vi "Optical Pulse Sequence Generator with ref pulse.vi"(6 "N Loop":i32=25000, 7 "Sig/Ref pause":dbl, 8 "AOM Rest time":dbl, 9 "Signal delay":dbl, 10 "APD signal width":dbl, 11 "AOM Pulse length":dbl=3e-07) -> (0 "Array":T1(array[cluster]), 3 "No. Instructions":i32)   [LabVIEW 2012]
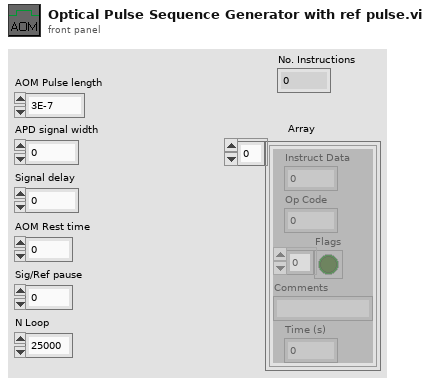
[diagram p1: front panel]
types:
  T1 = cluster{"Instruct Data":i32, "Op Code":i32, "Flags":bool[], "Comments":string, "Time (s)":dbl}[]
  T2 = cluster{"Instruct Data":i32, "Op Code":i32, "Flags":bool[], "Comments":string, "Time (s)":dbl}
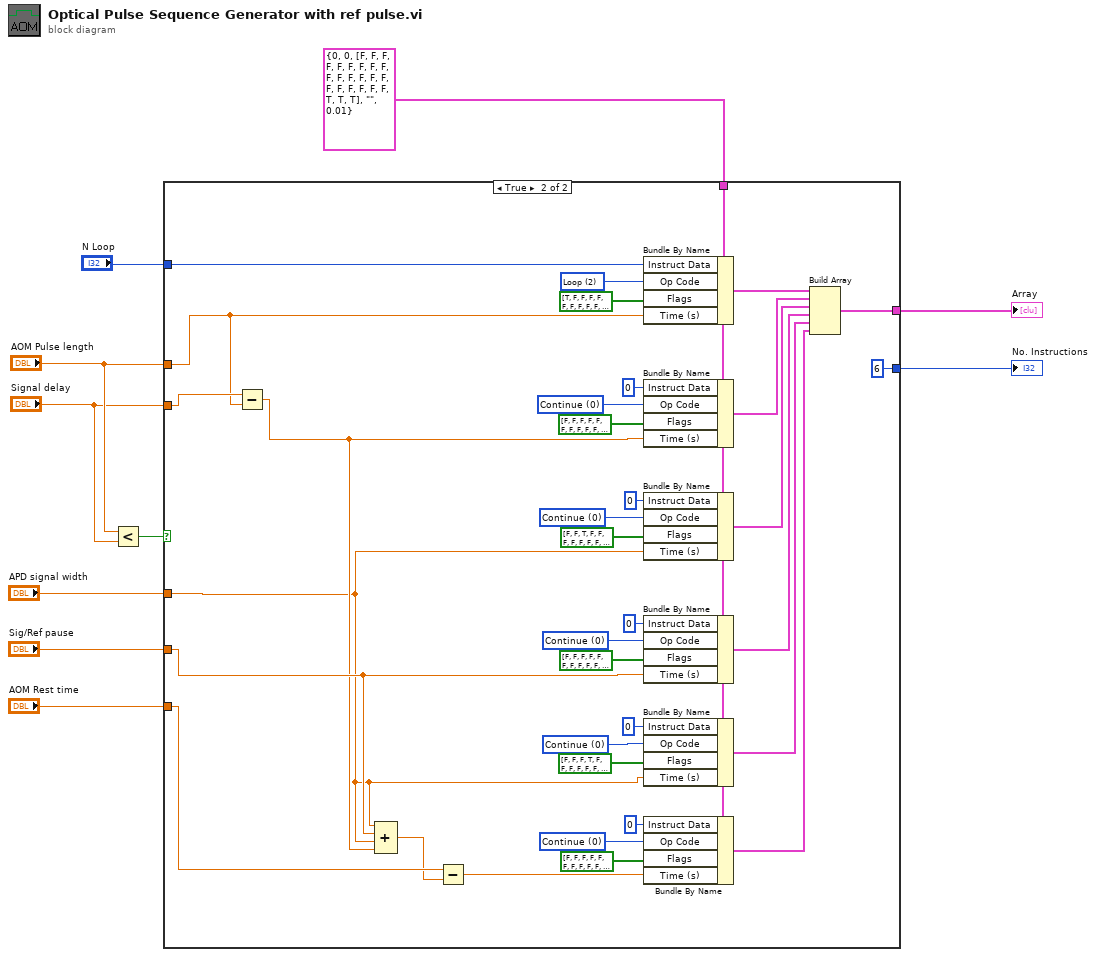
[diagram p0: block diagram]
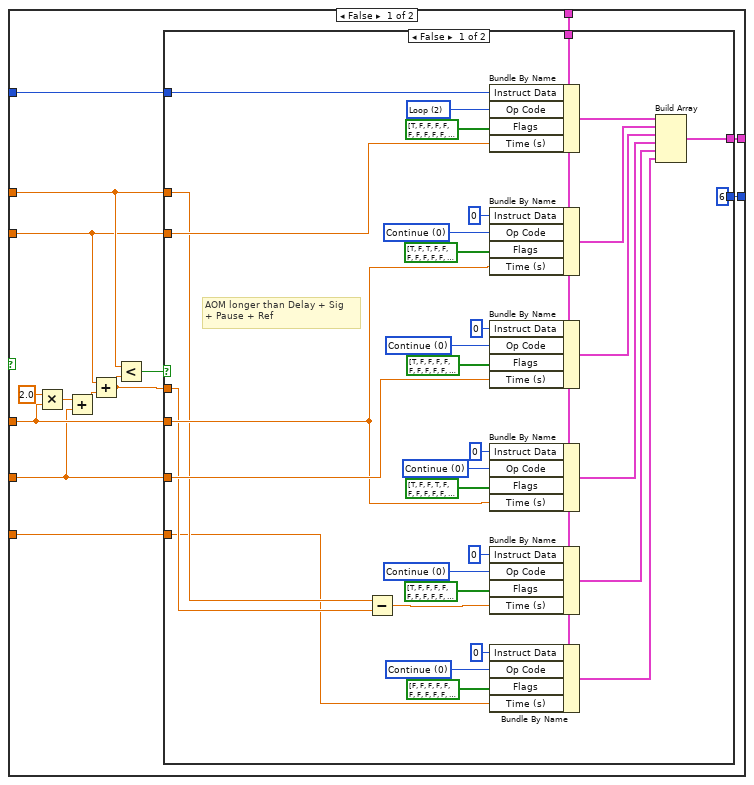
[diagram p2: hidden frame]
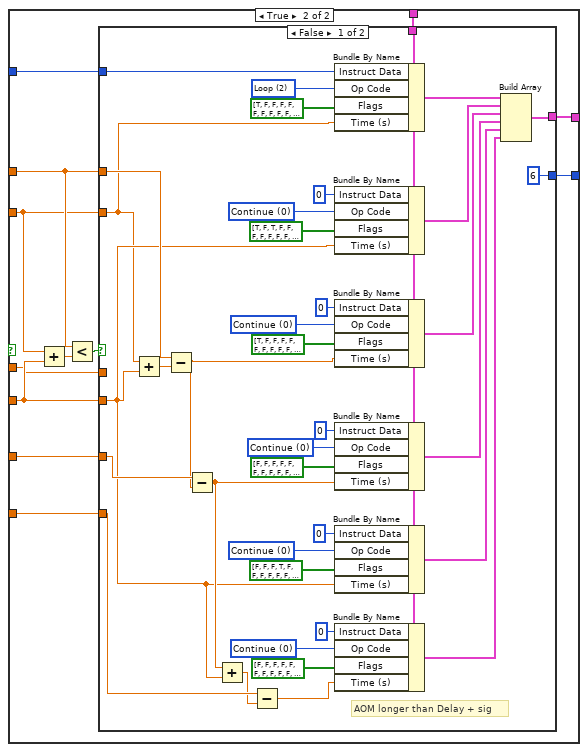
[diagram p3: hidden frame]
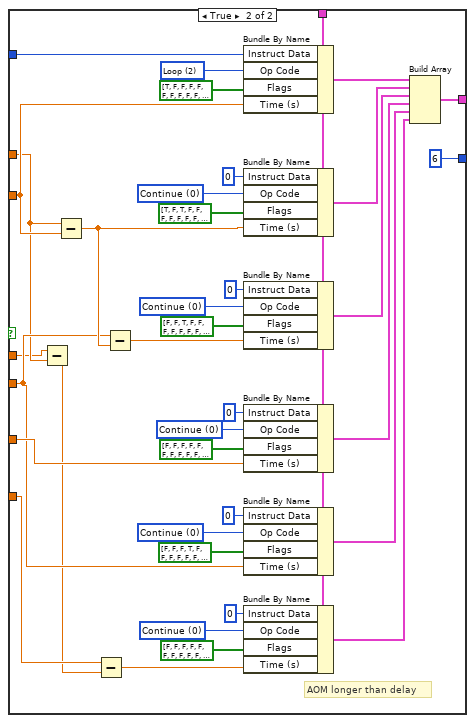
[diagram p4: hidden frame]
diagram:
  n1 = Less?(x="AOM Pulse length", y="Signal delay") -> (x < y?=w10:bool)
  n2 = case shown="True" w10 {
    tunnel: "AOM Pulse length" -> [w18 w145]
    tunnel: "Signal delay" -> [w17 w146]
    tunnel: "APD signal width" -> [w16 w151]
    tunnel: "AOM Rest time" -> [w14 w150]
    tunnel: "Sig/Ref pause" -> [w15 w153]
    tunnel: T2 {"Instruct Data"=0, "Op Code"=0, "Flags"=[FALSE, FALSE, FALSE, FALSE, FALSE, FALSE, FALSE, FALSE, FALSE, FALSE, FALSE, FALSE, FALSE, FALSE, FALSE, FALSE, FALSE, FALSE, FALSE, FALSE, FALSE, TRUE, TRUE, TRUE], "Comments"="", "Time (s)"=0.01} ("PB Inst 2") -> [w20 w155]
    tunnel: "N Loop" -> [w19 w156]
    tunnel: [w12 w154] -> w2
    tunnel: [w11 6] -> w1
    frame False {
      n3 = Multiply(x=2.0, y=w16) -> (x*y=w22:dbl)
      n4 = Add(x=w22, y=w15) -> (x+y=w21:dbl)
      n5 = Add(x=w17, y=w21) -> (x+y=w13:dbl)
      n6 = Less?(x=w18, y=w13) -> (x < y?=w24:bool)
      n7 = case shown="False" w24 {
        tunnel: w20 -> [w34 w65]
        tunnel: w19 -> [w56 w64]
        tunnel: w18 -> [w39 w69]
        tunnel: w17 -> [w55 w63]
        tunnel: w16 -> [w44 w60]
        tunnel: w15 -> [w48 w67]
        tunnel: w14 -> [w33 w66]
        tunnel: w13 -> [w40 w59]
        tunnel: [w26 w62] -> w12
        tunnel: [6 w61] -> w11
        frame False {
          w36 = 0 items=["Continue", "Stop", "Loop", "End Loop", "JSR", "RTS", "Branch", "Long Delay", "Wait"] ("Op Code")
          w42 = 0 items=["Continue", "Stop", "Loop", "End Loop", "JSR", "RTS", "Branch", "Long Delay", "Wait"] ("Op Code")
          w46 = 0 items=["Continue", "Stop", "Loop", "End Loop", "JSR", "RTS", "Branch", "Long Delay", "Wait"] ("Op Code")
          w50 = 0 items=["Continue", "Stop", "Loop", "End Loop", "JSR", "RTS", "Branch", "Long Delay", "Wait"] ("Op Code")
          w53 = 0 items=["Continue", "Stop", "Loop", "End Loop", "JSR", "RTS", "Branch", "Long Delay", "Wait"] ("Op Code")
          w57 = 2 items=["Continue", "Stop", "Loop", "End Loop", "JSR", "RTS", "Branch", "Long Delay", "Wait"] ("Op Code")
          # "AOM longer than Delay + Sig\n+ Pause + Ref"
          n8 = Subtract(x=w39, y=w40) -> (x-y=w38:dbl)
          n9 = Bundle By Name(cluster=w34, "Instruct Data"=w56, "Op Code"=w57, "Flags"=bool[] [TRUE, FALSE, FALSE, FALSE, FALSE, FALSE, FALSE, FALSE, FALSE, FALSE, FALSE, FALSE, FALSE, FALSE, FALSE, FALSE, FALSE, FALSE, FALSE, FALSE, FALSE, TRUE, TRUE, TRUE], "Time (s)"=w55) -> (w32:T2)
          n10 = Bundle By Name(cluster=w34, "Instruct Data"=0, "Op Code"=w53, "Flags"=bool[] [TRUE, FALSE, TRUE, FALSE, FALSE, FALSE, FALSE, FALSE, FALSE, FALSE, FALSE, FALSE, FALSE, FALSE, FALSE, FALSE, FALSE, FALSE, FALSE, FALSE, FALSE, TRUE, TRUE, TRUE], "Time (s)"=w44) -> (w27:T2)
          n11 = Bundle By Name(cluster=w34, "Instruct Data"=0, "Op Code"=w50, "Flags"=bool[] [TRUE, FALSE, FALSE, FALSE, FALSE, FALSE, FALSE, FALSE, FALSE, FALSE, FALSE, FALSE, FALSE, FALSE, FALSE, FALSE, FALSE, FALSE, FALSE, FALSE, FALSE, TRUE, TRUE, TRUE], "Time (s)"=w48) -> (w28:T2)
          n12 = Bundle By Name(cluster=w34, "Instruct Data"=0, "Op Code"=w46, "Flags"=bool[] [TRUE, FALSE, FALSE, TRUE, FALSE, FALSE, FALSE, FALSE, FALSE, FALSE, FALSE, FALSE, FALSE, FALSE, FALSE, FALSE, FALSE, FALSE, FALSE, FALSE, FALSE, TRUE, TRUE, TRUE], "Time (s)"=w44) -> (w29:T2)
          n13 = Bundle By Name(cluster=w34, "Instruct Data"=0, "Op Code"=w42, "Flags"=bool[] [TRUE, FALSE, FALSE, FALSE, FALSE, FALSE, FALSE, FALSE, FALSE, FALSE, FALSE, FALSE, FALSE, FALSE, FALSE, FALSE, FALSE, FALSE, FALSE, FALSE, FALSE, TRUE, TRUE, TRUE], "Time (s)"=w38) -> (w30:T2)
          n14 = Bundle By Name(cluster=w34, "Instruct Data"=0, "Op Code"=w36, "Flags"=bool[] [FALSE, FALSE, FALSE, FALSE, FALSE, FALSE, FALSE, FALSE, FALSE, FALSE, FALSE, FALSE, FALSE, FALSE, FALSE, FALSE, FALSE, FALSE, FALSE, FALSE, FALSE, TRUE, TRUE, TRUE], "Time (s)"=w33) -> (w31:T2)
          n15 = Build Array(w32, w27, w28, w29, w30, w31) -> (w26:T1)
        }
        frame True {
          n16 = Add(x=w63, y=w60) -> (x+y=w68:dbl)
          n17 = Less?(x=w69, y=w68) -> (x < y?=w70:bool)
          n18 = case shown="False" w70 {
            tunnel: w69 -> [w74 w113]
            tunnel: w60 -> [w72 w115]
            tunnel: w67 -> [w81 w116]
            tunnel: w66 -> [w78 w114]
            tunnel: w65 -> [w84 w121]
            tunnel: w64 -> [w82 w120]
            tunnel: w63 -> [w71 w119]
            tunnel: [w83 w110] -> w62
            tunnel: [6 6] -> w61
            tunnel: w59 -> [_ w108]
            frame False {
              w100 = 0 items=["Continue", "Stop", "Loop", "End Loop", "JSR", "RTS", "Branch", "Long Delay", "Wait"] ("Op Code")
              w97 = 0 items=["Continue", "Stop", "Loop", "End Loop", "JSR", "RTS", "Branch", "Long Delay", "Wait"] ("Op Code")
              w94 = 0 items=["Continue", "Stop", "Loop", "End Loop", "JSR", "RTS", "Branch", "Long Delay", "Wait"] ("Op Code")
              w91 = 0 items=["Continue", "Stop", "Loop", "End Loop", "JSR", "RTS", "Branch", "Long Delay", "Wait"] ("Op Code")
              w88 = 0 items=["Continue", "Stop", "Loop", "End Loop", "JSR", "RTS", "Branch", "Long Delay", "Wait"] ("Op Code")
              w86 = 2 items=["Continue", "Stop", "Loop", "End Loop", "JSR", "RTS", "Branch", "Long Delay", "Wait"] ("Op Code")
              # "AOM longer than Delay + sig"
              n19 = Add(x=w71, y=w72) -> (x+y=w73:dbl)
              n20 = Subtract(x=w74, y=w73) -> (x-y=w80:dbl)
              n21 = Subtract(x=w81, y=w80) -> (x-y=w79:dbl)
              n22 = Add(x=w79, y=w72) -> (x+y=w77:dbl)
              n23 = Subtract(x=w78, y=w77) -> (x-y=w76:dbl)
              n24 = Bundle By Name(cluster=w84, "Instruct Data"=w82, "Op Code"=w86, "Flags"=bool[] [TRUE, FALSE, FALSE, FALSE, FALSE, FALSE, FALSE, FALSE, FALSE, FALSE, FALSE, FALSE, FALSE, FALSE, FALSE, FALSE, FALSE, FALSE, FALSE, FALSE, FALSE, TRUE, TRUE, TRUE], "Time (s)"=w71) -> (w102:T2)
              n25 = Bundle By Name(cluster=w84, "Instruct Data"=0, "Op Code"=w88, "Flags"=bool[] [TRUE, FALSE, TRUE, FALSE, FALSE, FALSE, FALSE, FALSE, FALSE, FALSE, FALSE, FALSE, FALSE, FALSE, FALSE, FALSE, FALSE, FALSE, FALSE, FALSE, FALSE, TRUE, TRUE, TRUE], "Time (s)"=w72) -> (w107:T2)
              n26 = Bundle By Name(cluster=w84, "Instruct Data"=0, "Op Code"=w91, "Flags"=bool[] [TRUE, FALSE, FALSE, FALSE, FALSE, FALSE, FALSE, FALSE, FALSE, FALSE, FALSE, FALSE, FALSE, FALSE, FALSE, FALSE, FALSE, FALSE, FALSE, FALSE, FALSE, TRUE, TRUE, TRUE], "Time (s)"=w80) -> (w106:T2)
              n27 = Bundle By Name(cluster=w84, "Instruct Data"=0, "Op Code"=w94, "Flags"=bool[] [FALSE, FALSE, FALSE, FALSE, FALSE, FALSE, FALSE, FALSE, FALSE, FALSE, FALSE, FALSE, FALSE, FALSE, FALSE, FALSE, FALSE, FALSE, FALSE, FALSE, FALSE, TRUE, TRUE, TRUE], "Time (s)"=w79) -> (w105:T2)
              n28 = Bundle By Name(cluster=w84, "Instruct Data"=0, "Op Code"=w97, "Flags"=bool[] [FALSE, FALSE, FALSE, TRUE, FALSE, FALSE, FALSE, FALSE, FALSE, FALSE, FALSE, FALSE, FALSE, FALSE, FALSE, FALSE, FALSE, FALSE, FALSE, FALSE, FALSE, TRUE, TRUE, TRUE], "Time (s)"=w72) -> (w104:T2)
              n29 = Bundle By Name(cluster=w84, "Instruct Data"=0, "Op Code"=w100, "Flags"=bool[] [FALSE, FALSE, FALSE, FALSE, FALSE, FALSE, FALSE, FALSE, FALSE, FALSE, FALSE, FALSE, FALSE, FALSE, FALSE, FALSE, FALSE, FALSE, FALSE, FALSE, FALSE, TRUE, TRUE, TRUE], "Time (s)"=w76) -> (w103:T2)
              n30 = Build Array(w102, w107, w106, w105, w104, w103) -> (w83:T1)
            }
            frame True {
              w137 = 0 items=["Continue", "Stop", "Loop", "End Loop", "JSR", "RTS", "Branch", "Long Delay", "Wait"] ("Op Code")
              w134 = 0 items=["Continue", "Stop", "Loop", "End Loop", "JSR", "RTS", "Branch", "Long Delay", "Wait"] ("Op Code")
              w131 = 0 items=["Continue", "Stop", "Loop", "End Loop", "JSR", "RTS", "Branch", "Long Delay", "Wait"] ("Op Code")
              w128 = 0 items=["Continue", "Stop", "Loop", "End Loop", "JSR", "RTS", "Branch", "Long Delay", "Wait"] ("Op Code")
              w125 = 0 items=["Continue", "Stop", "Loop", "End Loop", "JSR", "RTS", "Branch", "Long Delay", "Wait"] ("Op Code")
              w123 = 2 items=["Continue", "Stop", "Loop", "End Loop", "JSR", "RTS", "Branch", "Long Delay", "Wait"] ("Op Code")
              # "AOM longer than delay"
              n31 = Subtract(x=w108, y=w113) -> (x-y=w112:dbl)
              n32 = Subtract(x=w113, y=w119) -> (x-y=w118:dbl)
              n33 = Subtract(x=w114, y=w112) -> (x-y=w111:dbl)
              n34 = Subtract(x=w115, y=w118) -> (x-y=w117:dbl)
              n35 = Bundle By Name(cluster=w121, "Instruct Data"=w120, "Op Code"=w123, "Flags"=bool[] [TRUE, FALSE, FALSE, FALSE, FALSE, FALSE, FALSE, FALSE, FALSE, FALSE, FALSE, FALSE, FALSE, FALSE, FALSE, FALSE, FALSE, FALSE, FALSE, FALSE, FALSE, TRUE, TRUE, TRUE], "Time (s)"=w119) -> (w139:T2)
              n36 = Bundle By Name(cluster=w121, "Instruct Data"=0, "Op Code"=w125, "Flags"=bool[] [TRUE, FALSE, TRUE, FALSE, FALSE, FALSE, FALSE, FALSE, FALSE, FALSE, FALSE, FALSE, FALSE, FALSE, FALSE, FALSE, FALSE, FALSE, FALSE, FALSE, FALSE, TRUE, TRUE, TRUE], "Time (s)"=w118) -> (w144:T2)
              n37 = Bundle By Name(cluster=w121, "Instruct Data"=0, "Op Code"=w128, "Flags"=bool[] [FALSE, FALSE, TRUE, FALSE, FALSE, FALSE, FALSE, FALSE, FALSE, FALSE, FALSE, FALSE, FALSE, FALSE, FALSE, FALSE, FALSE, FALSE, FALSE, FALSE, FALSE, TRUE, TRUE, TRUE], "Time (s)"=w117) -> (w143:T2)
              n38 = Bundle By Name(cluster=w121, "Instruct Data"=0, "Op Code"=w131, "Flags"=bool[] [FALSE, FALSE, FALSE, FALSE, FALSE, FALSE, FALSE, FALSE, FALSE, FALSE, FALSE, FALSE, FALSE, FALSE, FALSE, FALSE, FALSE, FALSE, FALSE, FALSE, FALSE, TRUE, TRUE, TRUE], "Time (s)"=w116) -> (w142:T2)
              n39 = Bundle By Name(cluster=w121, "Instruct Data"=0, "Op Code"=w134, "Flags"=bool[] [FALSE, FALSE, FALSE, TRUE, FALSE, FALSE, FALSE, FALSE, FALSE, FALSE, FALSE, FALSE, FALSE, FALSE, FALSE, FALSE, FALSE, FALSE, FALSE, FALSE, FALSE, TRUE, TRUE, TRUE], "Time (s)"=w115) -> (w141:T2)
              n40 = Bundle By Name(cluster=w121, "Instruct Data"=0, "Op Code"=w137, "Flags"=bool[] [FALSE, FALSE, FALSE, FALSE, FALSE, FALSE, FALSE, FALSE, FALSE, FALSE, FALSE, FALSE, FALSE, FALSE, FALSE, FALSE, FALSE, FALSE, FALSE, FALSE, FALSE, TRUE, TRUE, TRUE], "Time (s)"=w111) -> (w140:T2)
              n41 = Build Array(w139, w144, w143, w142, w141, w140) -> (w110:T1)
            }
          }
        }
      }
    }
    frame True {
      w172 = 0 items=["Continue", "Stop", "Loop", "End Loop", "JSR", "RTS", "Branch", "Long Delay", "Wait"] ("Op Code")
      w169 = 0 items=["Continue", "Stop", "Loop", "End Loop", "JSR", "RTS", "Branch", "Long Delay", "Wait"] ("Op Code")
      w166 = 0 items=["Continue", "Stop", "Loop", "End Loop", "JSR", "RTS", "Branch", "Long Delay", "Wait"] ("Op Code")
      w163 = 0 items=["Continue", "Stop", "Loop", "End Loop", "JSR", "RTS", "Branch", "Long Delay", "Wait"] ("Op Code")
      w160 = 0 items=["Continue", "Stop", "Loop", "End Loop", "JSR", "RTS", "Branch", "Long Delay", "Wait"] ("Op Code")
      w158 = 2 items=["Continue", "Stop", "Loop", "End Loop", "JSR", "RTS", "Branch", "Long Delay", "Wait"] ("Op Code")
      n42 = Subtract(x=w146, y=w145) -> (x-y=w152:dbl)
      n43 = Compound Arithmetic op=ADD(w151, w153, w151, w152) -> (w149:dbl)
      n44 = Subtract(x=w150, y=w149) -> (x-y=w148:dbl)
      n45 = Bundle By Name(cluster=w155, "Instruct Data"=w156, "Op Code"=w158, "Flags"=bool[] [TRUE, FALSE, FALSE, FALSE, FALSE, FALSE, FALSE, FALSE, FALSE, FALSE, FALSE, FALSE, FALSE, FALSE, FALSE, FALSE, FALSE, FALSE, FALSE, FALSE, FALSE, TRUE, TRUE, TRUE], "Time (s)"=w145) -> (w174:T2)
      n46 = Bundle By Name(cluster=w155, "Instruct Data"=0, "Op Code"=w160, "Flags"=bool[] [FALSE, FALSE, FALSE, FALSE, FALSE, FALSE, FALSE, FALSE, FALSE, FALSE, FALSE, FALSE, FALSE, FALSE, FALSE, FALSE, FALSE, FALSE, FALSE, FALSE, FALSE, TRUE, TRUE, TRUE], "Time (s)"=w152) -> (w179:T2)
      n47 = Bundle By Name(cluster=w155, "Instruct Data"=0, "Op Code"=w163, "Flags"=bool[] [FALSE, FALSE, TRUE, FALSE, FALSE, FALSE, FALSE, FALSE, FALSE, FALSE, FALSE, FALSE, FALSE, FALSE, FALSE, FALSE, FALSE, FALSE, FALSE, FALSE, FALSE, TRUE, TRUE, TRUE], "Time (s)"=w151) -> (w178:T2)
      n48 = Bundle By Name(cluster=w155, "Instruct Data"=0, "Op Code"=w166, "Flags"=bool[] [FALSE, FALSE, FALSE, FALSE, FALSE, FALSE, FALSE, FALSE, FALSE, FALSE, FALSE, FALSE, FALSE, FALSE, FALSE, FALSE, FALSE, FALSE, FALSE, FALSE, FALSE, TRUE, TRUE, TRUE], "Time (s)"=w153) -> (w177:T2)
      n49 = Bundle By Name(cluster=w155, "Instruct Data"=0, "Op Code"=w169, "Flags"=bool[] [FALSE, FALSE, FALSE, TRUE, FALSE, FALSE, FALSE, FALSE, FALSE, FALSE, FALSE, FALSE, FALSE, FALSE, FALSE, FALSE, FALSE, FALSE, FALSE, FALSE, FALSE, TRUE, TRUE, TRUE], "Time (s)"=w151) -> (w176:T2)
      n50 = Bundle By Name(cluster=w155, "Instruct Data"=0, "Op Code"=w172, "Flags"=bool[] [FALSE, FALSE, FALSE, FALSE, FALSE, FALSE, FALSE, FALSE, FALSE, FALSE, FALSE, FALSE, FALSE, FALSE, FALSE, FALSE, FALSE, FALSE, FALSE, FALSE, FALSE, TRUE, TRUE, TRUE], "Time (s)"=w148) -> (w175:T2)
      n51 = Build Array(w174, w179, w178, w177, w176, w175) -> (w154:T1)
    }
  }
  "Array" <- w2
  "No. Instructions" <- w1
